vi "Add Offsets.vi"(4 "Cluster":T2, 5 "RR Data":T1, 6 "RL Data":T1, 7 "FL Data":T1, 8 "FR Data":T1) -> (0 "RR Data Out":T1, 1 "RL Data Out":T1, 2 "FL Data Out":T1, 3 "FR Data Out":T1)   [LabVIEW 2018]
uses:
  Angle offsets.ctl
  Final Motor Data.ctl
  <vilib>/Rock Robotics/Network Tables/NT Write Number.vi
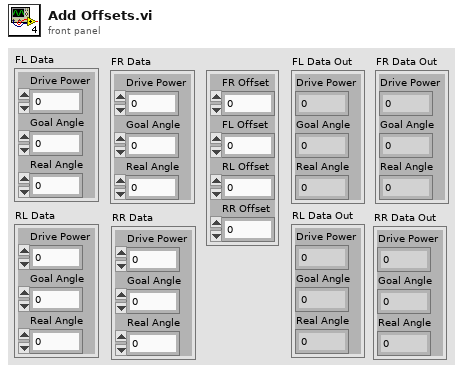
[diagram p1: front panel]
types:
  T1 = typedef "Final Motor Data.ctl" = cluster{"Drive Power":dbl, "Goal Angle":dbl, "Real Angle":dbl}
  T2 = typedef "Angle offsets.ctl" = cluster{"FR Offset":dbl, "FL Offset":dbl, "RL Offset":dbl, "RR Offset":dbl}
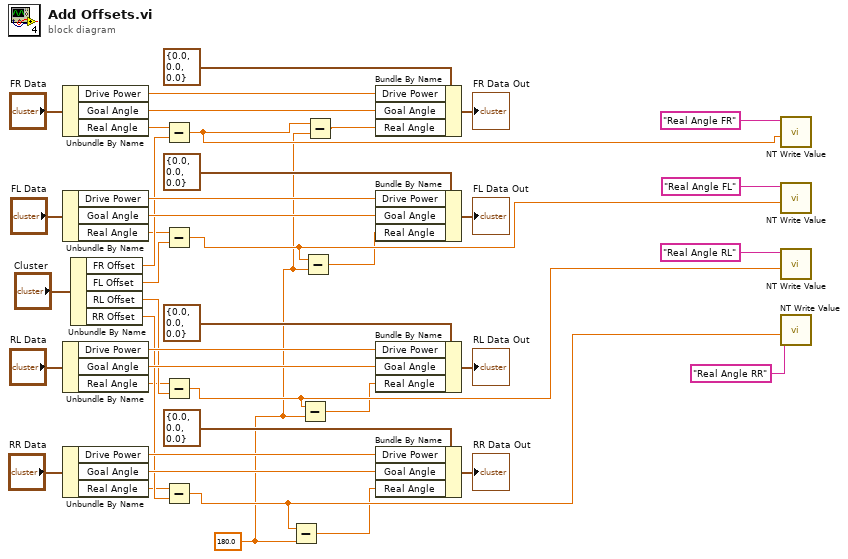
[diagram p0: block diagram]
diagram:
  w1 = 180.0
  n1 = Unbundle By Name("FR Data") -> ("Drive Power"=w28:dbl, "Goal Angle"=w29:dbl, "Real Angle"=w20:dbl)
  n2 = Unbundle By Name("FL Data") -> ("Drive Power"=w27:dbl, "Goal Angle"=w26:dbl, "Real Angle"=w16:dbl)
  n3 = Unbundle By Name("RL Data") -> ("Drive Power"=w25:dbl, "Goal Angle"=w24:dbl, "Real Angle"=w15:dbl)
  n4 = Unbundle By Name("RR Data") -> ("Drive Power"=w23:dbl, "Goal Angle"=w22:dbl, "Real Angle"=w14:dbl)
  n5 = Unbundle By Name("Cluster") -> ("FR Offset"=w21:dbl, "FL Offset"=w19:dbl, "RL Offset"=w18:dbl, "RR Offset"=w17:dbl)
  n6 = Subtract(x=w20, y=w21) -> (x-y=w9:dbl)
  n7 = Subtract(x=w16, y=w19) -> (x-y=w7:dbl)
  n8 = Subtract(x=w15, y=w18) -> (x-y=w5:dbl)
  n9 = Subtract(x=w14, y=w17) -> (x-y=w3:dbl)
  n10 = Subtract(x=w3, y=w1) -> (x-y=w2:dbl)
  n11 = Subtract(x=w5, y=w1) -> (x-y=w4:dbl)
  n12 = Subtract(x=w7, y=w1) -> (x-y=w6:dbl)
  n13 = Subtract(x=w9, y=w1) -> (x-y=w8:dbl)
  n14 = Bundle By Name(cluster=T1 {"Drive Power"=0.0, "Goal Angle"=0.0, "Real Angle"=0.0} ("FR Data Out 2"), "Drive Power"=w28, "Goal Angle"=w29, "Real Angle"=w8) -> (→"FR Data Out":T1)
  n15 = Bundle By Name(cluster=T1 {"Drive Power"=0.0, "Goal Angle"=0.0, "Real Angle"=0.0} ("FL Data Out 2"), "Drive Power"=w27, "Goal Angle"=w26, "Real Angle"=w6) -> (→"FL Data Out":T1)
  n16 = Bundle By Name(cluster=T1 {"Drive Power"=0.0, "Goal Angle"=0.0, "Real Angle"=0.0} ("RL Data Out 2"), "Drive Power"=w25, "Goal Angle"=w24, "Real Angle"=w4) -> (→"RL Data Out":T1)
  n17 = Bundle By Name(cluster=T1 {"Drive Power"=0.0, "Goal Angle"=0.0, "Real Angle"=0.0} ("RR Data Out 2"), "Drive Power"=w23, "Goal Angle"=w22, "Real Angle"=w2) -> (→"RR Data Out":T1)
  n18 = call-poly <vilib>:"NT Write Value.vi"("Numeric"=w9, "Name"="Real Angle FR") -> ()  [unwired: 9 in, 1 out]
  n19 = call-poly <vilib>:"NT Write Value.vi"("Numeric"=w7, "Name"="Real Angle FL") -> ()  [unwired: 9 in, 1 out]
  n20 = call-poly <vilib>:"NT Write Value.vi"("Numeric"=w5, "Name"="Real Angle RL") -> ()  [unwired: 9 in, 1 out]
  n21 = call-poly <vilib>:"NT Write Value.vi"("Numeric"=w3, "Name"="Real Angle RR") -> ()  [unwired: 9 in, 1 out]
